vi "LoadConf.vi"(8 "error in":errorcluster, 10 "MEC":string, 11 "Controlador in":refnum<class "Controlador.lvclass">) -> (0 "error out":errorcluster, 3 "Controlador out":refnum<class "Controlador.lvclass">)   [LabVIEW 2018, in "Controlador.lvclass"]
uses:
  Controlador.lvclass
  Controlador.lvclass/Controlador.ctl
  Global Coude.vi
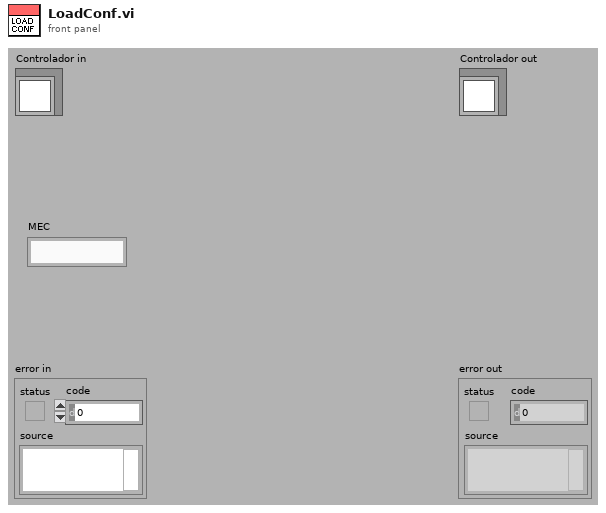
[diagram p1: front panel]
types:
  T1 = cluster{"Mec ID":string, "VISA Mec":refnum<visa-resource-name>, "Mec PosLimit":string, "Mec NegLimit":string, "MecOffset":string, "MecTargets":dbl[], "MecEnabled":bool, "Mec Target":dbl}
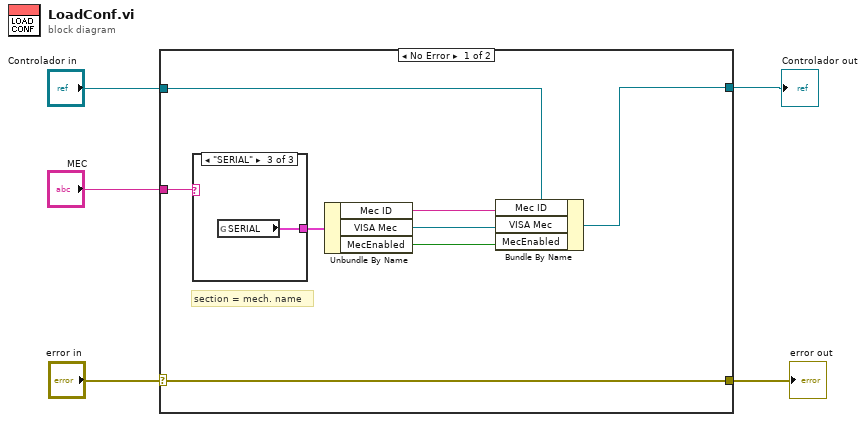
[diagram p0: block diagram]
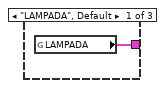
[diagram p2: hidden frame]
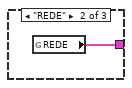
[diagram p3: hidden frame]
diagram:
  n1 = case shown="No Error" "error in" {
    selector: "error in" -> [w6 w18]
    tunnel: [w6 w18] -> w2
    tunnel: [w11 w17] -> w1
    tunnel: "Controlador in" -> [w10 w17]
    tunnel: "MEC" -> [w13 _]
    frame No Error {
      # "section = mech. name"
      n2 = case shown="\"SERIAL\"" w13 {
        tunnel: [w14 w15 w16] -> w12
        frame "LAMPADA", Default {
          n3 = global read "Global Coude.vi" "LAMPADA"() -> (w14:T1)
        }
        frame "REDE" {
          n4 = global read "Global Coude.vi" "REDE"() -> (w15:T1)
        }
        frame "SERIAL" {
          n5 = global read "Global Coude.vi" "SERIAL"() -> (w16:T1)
        }
      }
      n6 = Unbundle By Name(w12) -> ("Mec ID"=w9:string, "VISA Mec"=w8:refnum<visa-resource-name>, "MecEnabled"=w7:bool)
      n7 = Bundle By Name(cluster=w10, "Mec ID"=w9, "VISA Mec"=w8, "MecEnabled"=w7) -> (w11:refnum<class "Controlador.lvclass">)
    }
    frame Error {
    }
  }
  "error out" <- w2
  "Controlador out" <- w1
